vi "Generic file paths.vi"(8 "error in (no error)":errorcluster, 11 "Parent Folder":path=path "G:/My Drive/Nanosurf_data_processing/Nanosurf_data") -> (0 "error out":errorcluster, 1 "SVG Path":string, 2 "BMP for inkscape path":string, 3 "BMP Path":string)   [LabVIEW 2016]
panel:
  out "result string":string
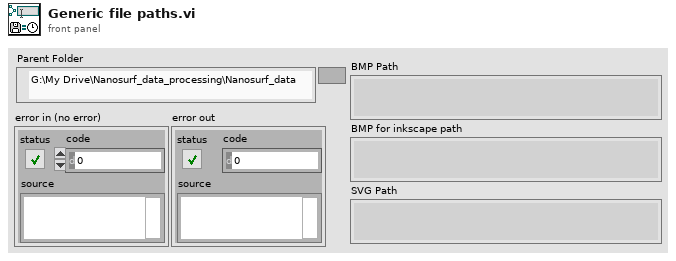
[diagram p1: front panel]
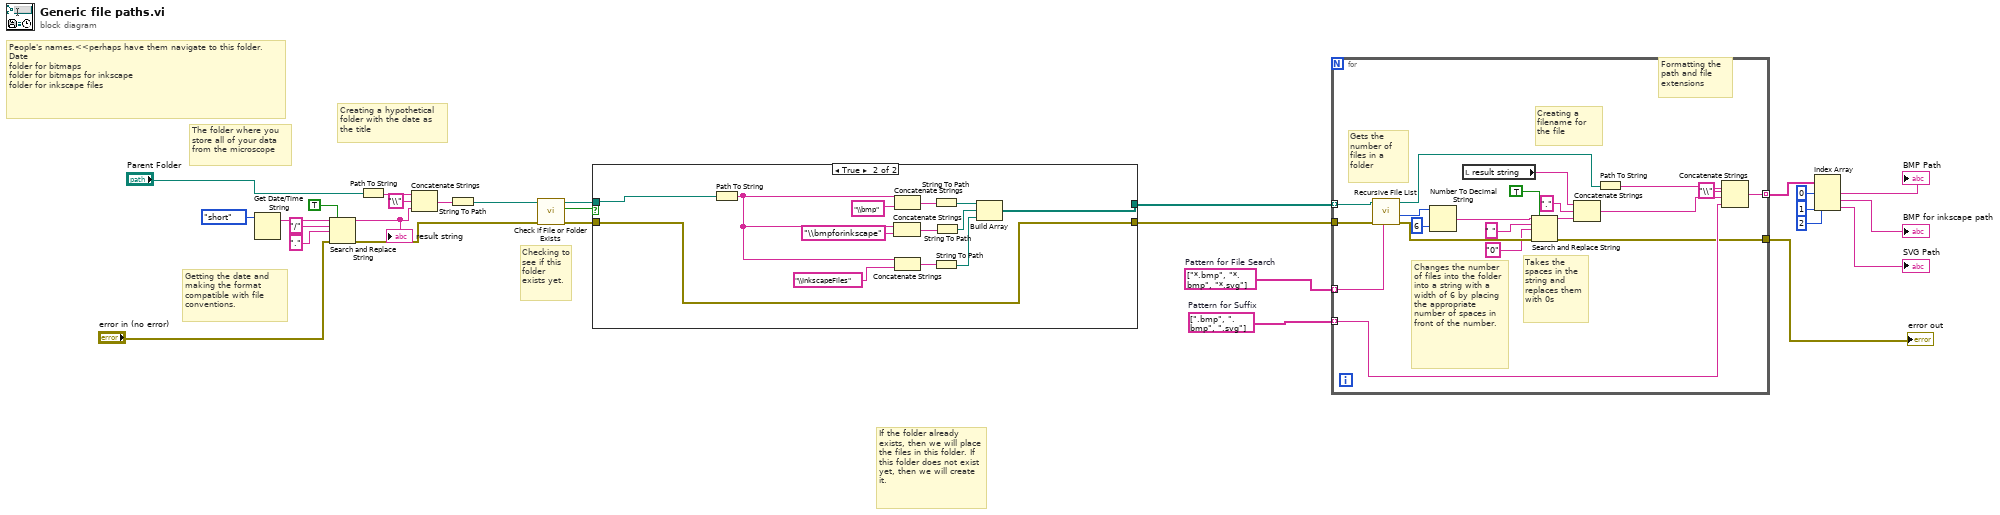
[diagram p0: block diagram]
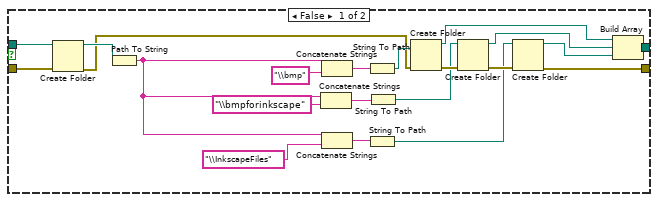
[diagram p2: hidden frame]
diagram:
  w9 = string[] ["*.bmp", "*.bmp", "*.svg"]  # Pattern for File Search
  w10 = string[] [".bmp", ".bmp", ".svg"]  # Pattern for Suffix
  # "Checking to see if this folder exists yet."
  # "Creating a hypothetical folder with the date as the title"
  # "Getting the date and making the format compatible with file conventions."
  # "The folder where you store all of your data from the microscope"
  # "If the folder already exists, then we will place the files in this folder. If this folder does not exist yet, then we will create it."
  # "People's names.<<perhaps have them navigate to this folder.\nDate\nfolder for bitmaps\nfolder for bitmaps for inkscape\nfolder for inkscape files"
  n1 = Get Date/Time String(date format (0)=enum16{"short", "long", "abbreviated"}."short") -> (date string=w24:string)  [unwired: 2 in, 1 out]
  n2 = Search and Replace String(replace all?=TRUE ("replace all? (F)"), input string=w24, search string="/", replace string="." ("replace string (\"\")"), error in="error in (no error)") -> (result string=w15:string, error out=w17:errorcluster)  [unwired: 3 in, 2 out]
  "result string" <- w15
  n3 = Path To String(path="Parent Folder") -> (string=w21:string)
  n4 = Concatenate Strings(w21, "\\" ("string"), w15) -> (w19:string)
  n5 = String To Path(string=w19) -> (path=w18:path)
  n6 = call <vilib>:"Check if File or Folder Exists.vi"("error in (no error)"=w17, "path"=w18) -> ("error out"=w26:errorcluster, "file or folder exists?"=w27:bool, "dup path"=w28:path)  [unwired: 7 in]
  n7 = case shown="True" w27 {
    tunnel: w28 -> [w49 w54]
    tunnel: w26 -> [w48 w55]
    tunnel: [w37 w55] -> w16
    tunnel: [w29 w50] -> w11
    frame False {
      n8 = Create Folder(path (use dialog)=w49, error in=w48) -> (created path=w47:path, error out=w33:errorcluster)  [unwired: 1 in, 1 out]
      n9 = Path To String(path=w47) -> (string=w45:string)
      n10 = Concatenate Strings(w45, "\\bmpforinkscape" ("string")) -> (w41:string)
      n11 = Concatenate Strings(w45, "\\bmp" ("string")) -> (w42:string)
      n12 = Concatenate Strings(w45, "\\InkscapeFiles" ("string")) -> (w40:string)
      n13 = String To Path(string=w42) -> (path=w36:path)
      n14 = String To Path(string=w40) -> (path=w34:path)
      n15 = String To Path(string=w41) -> (path=w35:path)
      n16 = Create Folder(path (use dialog)=w36, error in=w33) -> (created path=w30:path, error out=w38:errorcluster)  [unwired: 1 in, 1 out]
      n17 = Create Folder(path (use dialog)=w35, error in=w38) -> (created path=w32:path, error out=w39:errorcluster)  [unwired: 1 in, 1 out]
      n18 = Create Folder(path (use dialog)=w34, error in=w39) -> (created path=w31:path, error out=w37:errorcluster)  [unwired: 1 in, 1 out]
      n19 = Build Array(w30, w32, w31) -> (w29:path[])
    }
    frame True {
      n20 = Path To String(path=w54) -> (string=w61:string)
      n21 = Concatenate Strings(w61, "\\bmpforinkscape" ("string")) -> (w57:string)
      n22 = Concatenate Strings(w61, "\\bmp" ("string")) -> (w58:string)
      n23 = Concatenate Strings(w61, "\\InkscapeFiles" ("string")) -> (w56:string)
      n24 = String To Path(string=w58) -> (path=w53:path)
      n25 = String To Path(string=w56) -> (path=w51:path)
      n26 = String To Path(string=w57) -> (path=w52:path)
      n27 = Build Array(w53, w52, w51) -> (w50:path[])
    }
  }
  n28 = for {
    tunnel: w16 -> [w82]
    tunnel: w11 -> [w68] mode=indexing
    tunnel: w10 -> [w66] mode=indexing
    tunnel: [w65] -> w8 mode=indexing
    tunnel: w9 -> [w64] mode=indexing
    tunnel: [w63] -> w1
    # "Formatting the path and file extensions"
    # "Creating a filename for the file"
    # "Takes the spaces in the string and replaces them with 0s"
    # "Changes the number of files into the folder into a string with a width of 6 by placing the appropriate number of spaces in front of the number."
    # "Gets the number of files in a folder"
    n29 = call <vilib>:"Recursive File List.vi"("pattern"=w64, "error in (no error)"=w82, "Folder Path"=w68) -> ("error out"=w74:errorcluster, "Number of Files"=w71:i32, "dup Folder Path"=w72:path)  [unwired: 4 in, 2 out]
    n30 = Number To Decimal String(number=w71, width (-)=i16 6) -> (decimal integer string=w80:string)
    n31 = local read "result string"() -> (w75:string)
    n32 = Search and Replace String(replace all?=TRUE ("replace all? (F)"), input string=w80, search string=" ", replace string="0" ("replace string (\"\")"), error in=w74) -> (result string=w78:string, error out=w63:errorcluster)  [unwired: 3 in, 2 out]
    n33 = Concatenate Strings(w75, "." ("string"), w78) -> (w69:string)
    n34 = Path To String(path=w72) -> (string=w70:string)
    n35 = Concatenate Strings(w70, "\\" ("string"), w69, w66) -> (w65:string)
  }
  "error out" <- w1
  n36 = Index Array(array=w8, index #1=0 ("index"), index #2=1 ("index"), index #3=2 ("index")) -> (element #1=→"BMP Path":string, element #2=→"BMP for inkscape path":string, element #3=→"SVG Path":string)
